vi "segundo.vi"   [LabVIEW 2012]
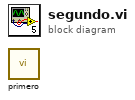
[diagram p0: block diagram]
diagram:
  n1 = call "primero.vi"() -> ()  [unwired: 3 in, 2 out]
